vi "Data Type to Assert 1D.vi"(8 "error in (no error)":errorcluster, 11 "Data Type":refnum<class "Data Type.lvclass">) -> (0 "error out":errorcluster, 3 "Assert 1D out":refnum<class "Assert.lvclass">[](array[class]))   [LabVIEW 2020, in "Assertion 1D.lvclass"]
uses:
  <vilib>/gpm_packages/@cs/data-type-serializer/source/Assertion 1D/Assertion 1D.lvclass
  <vilib>/gpm_packages/@cs/data-type-serializer/source/Data Type/Data Type.lvclass
  <vilib>/gpm_packages/@cs/run-time-assertions/Source/Assert/Assert.lvclass
  <vilib>/gpm_packages/@cs/data-type-serializer/source/Assertion 1D/Assertion 1D.lvclass/Assertion 1D.ctl
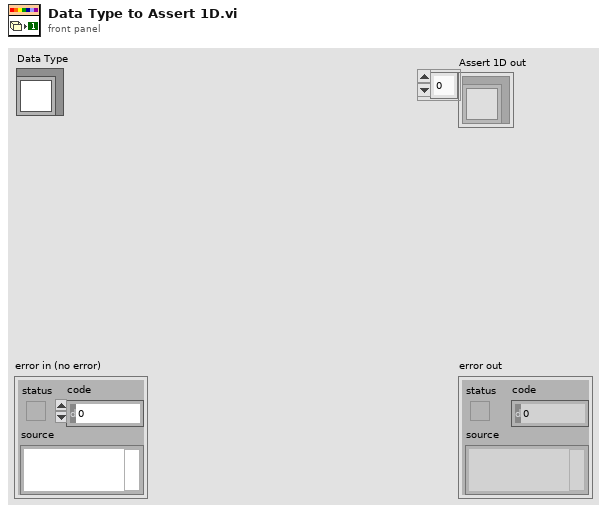
[diagram p1: front panel]
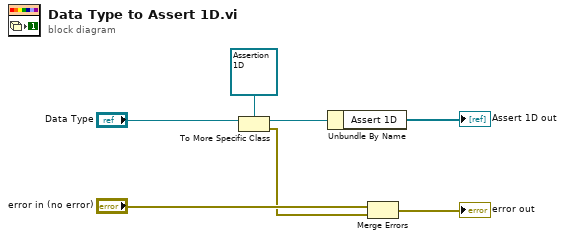
[diagram p0: block diagram]
diagram:
  n1 = To More Specific Class(target class=refnum<class "Assertion 1D.lvclass"> refnum ("Boolean out"), reference="Data Type") -> (specific class reference=w4:refnum<class "Assertion 1D.lvclass">, error out=w2:errorcluster)  [unwired: 1 in]
  n2 = Unbundle By Name(w4) -> ("Assert 1D"=→"Assert 1D out":refnum<class "Assert.lvclass">[])
  n3 = Merge Errors("error in (no error)", w2) -> (→"error out":errorcluster)
